vi "Map Complex Loopback to VS Channels.vi"(11 "Base Path to Ports":string) -> (2 "Rx Channel Array":string[](array[string]), 3 "Tx Channel Array":string[](array[string]))   [LabVIEW 2020, in "Single Core Complex Loopback.lvclass"]
uses:
  Single Core Complex Loopback.lvclass
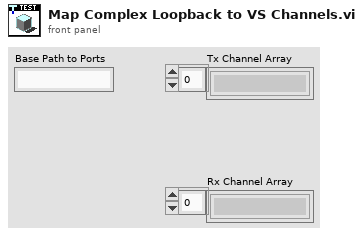
[diagram p1: front panel]
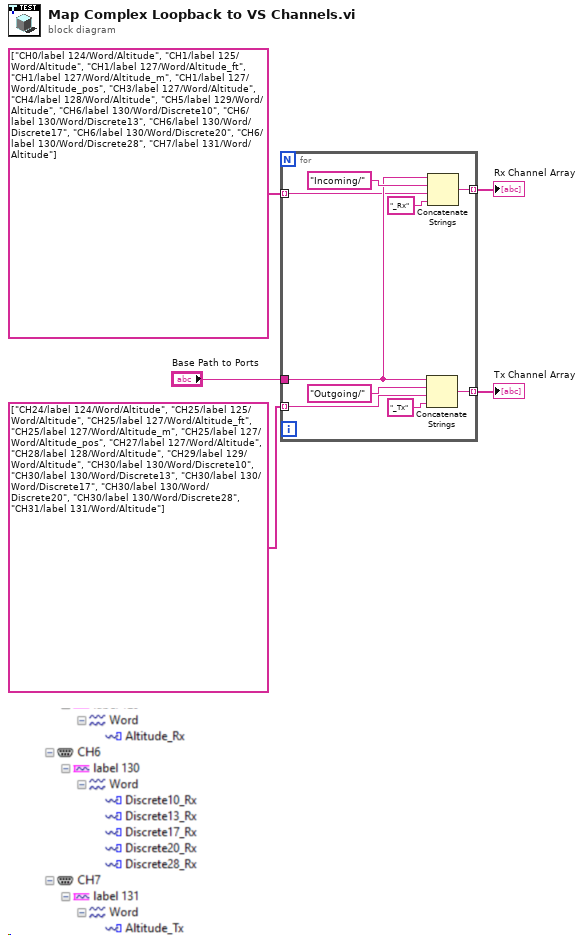
[diagram p0: block diagram]
diagram:
  n1 = for {
    tunnel: "Base Path to Ports" -> [w9]
    tunnel: string[] ["CH24/label 124/Word/Altitude", "CH25/label 125/Word/Altitude", "CH25/label 127/Word/Altitude_ft", "CH25/label 127/Word/Altitude_m", "CH25/label 127/Word/Altitude_pos", "CH27/label 127/Word/Altitude", "CH28/label 128/Word/Altitude", "CH29/label 129/Word/Altitude", "CH30/label 130/Word/Discrete10", "CH30/label 130/Word/Discrete13", "CH30/label 130/Word/Discrete17", "CH30/label 130/Word/Discrete20", "CH30/label 130/Word/Discrete28", "CH31/label 131/Word/Altitude"] -> [w14] mode=indexing
    tunnel: string[] ["CH0/label 124/Word/Altitude", "CH1/label 125/Word/Altitude", "CH1/label 127/Word/Altitude_ft", "CH1/label 127/Word/Altitude_m", "CH1/label 127/Word/Altitude_pos", "CH3/label 127/Word/Altitude", "CH4/label 128/Word/Altitude", "CH5/label 129/Word/Altitude", "CH6/label 130/Word/Discrete10", "CH6/label 130/Word/Discrete13", "CH6/label 130/Word/Discrete17", "CH6/label 130/Word/Discrete20", "CH6/label 130/Word/Discrete28", "CH7/label 131/Word/Altitude"] -> [w8] mode=indexing
    tunnel: [w13] -> w4 mode=indexing
    tunnel: [w12] -> w3 mode=indexing
    n2 = Concatenate Strings(w9, "Outgoing/" ("string"), w14, "_Tx" ("string")) -> (w12:string)
    n3 = Concatenate Strings(w9, "Incoming/" ("string"), w8, "_Rx" ("string")) -> (w13:string)
  }
  "Rx Channel Array" <- w4
  "Tx Channel Array" <- w3
